vi "Add.vi"(6 "Priority Message":bool, 7 "Q Ref In":refnum<queue>, 8 "error in":errorcluster, 10 "Payload":variant, 11 "Packet ID":string) -> (0 "error out":errorcluster, 5 "Q Ref Out":refnum<queue>)   [LabVIEW 2025, in "Q Wrappers.lvlib"]
uses:
  Q Wrappers.lvlib
  Q Packet.ctl
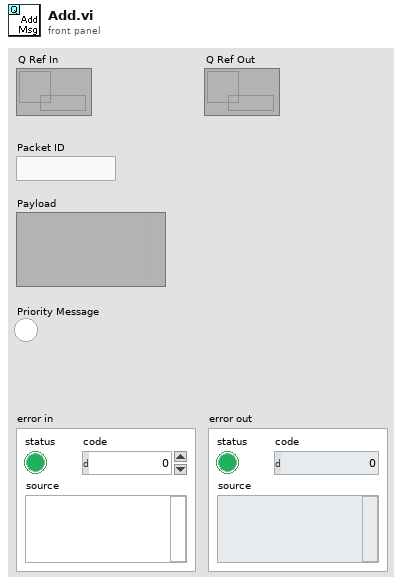
[diagram p1: front panel]
types:
  T1 = typedef "Q Packet.ctl" = cluster{"Packet ID":string, "Payload":variant}
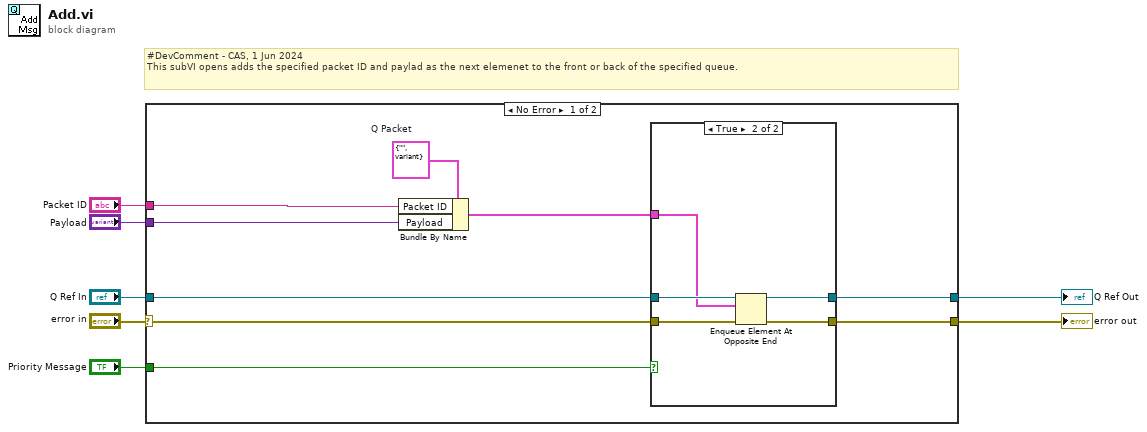
[diagram p0: block diagram]
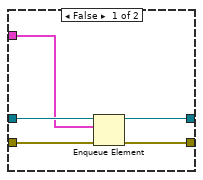
[diagram p2: hidden frame]
diagram:
  # "#DevComment - CAS, 1 Jun 2024\nThis subVI opens adds the specified packet ID and paylad as the next elemenet to the front or back of the specified queue."
  n1 = case shown="No Error" "error in" {
    selector: "error in" -> [w16 w27]
    tunnel: [w15 w27] -> w6
    tunnel: [w14 _] -> w5
    tunnel: "Q Ref In" -> [w12 _]
    tunnel: "Packet ID" -> [w11 _]
    tunnel: "Payload" -> [w10 _]
    tunnel: "Priority Message" -> [w8 _]
    frame No Error {
      w13 = T1 {"Packet ID"="", "Payload"=variant}  # Q Packet
      n2 = Bundle By Name(cluster=w13, "Packet ID"=w11, "Payload"=w10) -> (w9:T1)
      n3 = case shown="True" w8 {
        tunnel: w16 -> [w21 w26]
        tunnel: [w20 w25] -> w15
        tunnel: [w19 w24] -> w14
        tunnel: w12 -> [w18 w23]
        tunnel: w9 -> [w17 w22]
        frame False {
          n4 = Enqueue Element(queue=w18, element=w17, error in (no error)=w21) -> (queue out=w19:refnum<queue>, error out=w20:errorcluster)  [unwired: 1 in, 1 out]
        }
        frame True {
          n5 = Enqueue Element At Opposite End(queue=w23, element=w22, error in (no error)=w26) -> (queue out=w24:refnum<queue>, error out=w25:errorcluster)  [unwired: 1 in, 1 out]
        }
      }
    }
    frame Error {
    }
  }
  "error out" <- w6
  "Q Ref Out" <- w5
